vi "wfm_feature clear_adjunct.vi"(8 "error in (no error)":errorcluster, 11 "wfm_feature in":refnum<class "wfm_feature.lvclass">) -> (0 "error out":errorcluster, 3 "wfm_feature out":refnum<class "wfm_feature.lvclass">)   [LabVIEW 2018, in "wfm_feature.lvclass"]
uses:
  wfm_feature.lvclass
  wfm_feature.lvclass/wfm_feature.ctl
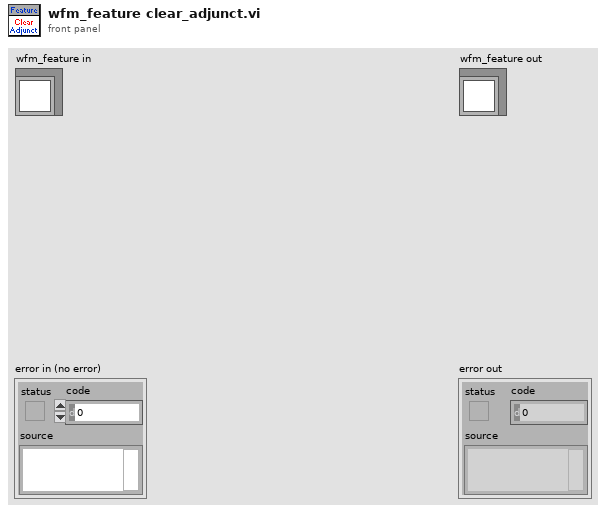
[diagram p1: front panel]
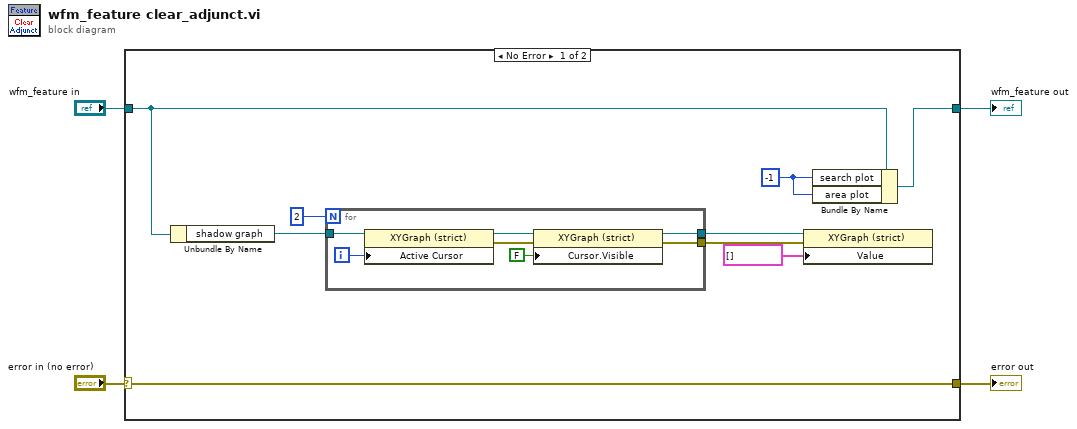
[diagram p0: block diagram]
diagram:
  n1 = case shown="No Error" "error in (no error)" {
    selector: "error in (no error)" -> [w13 w22]
    tunnel: [w13 w22] -> w3
    tunnel: [w5 w21] -> w1
    tunnel: "wfm_feature in" -> [w7 w21]
    frame No Error {
      w6 = -1 ("threshold plot")
      n2 = Unbundle By Name(w7) -> ("shadow graph"=w11:refnum<vi>)
      n3 = for {
        N: 2 -> [_]
        tunnel: w11 -> [w20]
        tunnel: [w15] -> w10
        tunnel: [w14] -> w9
        i -> [w19]
        n4 = property class="XYGraph (strict)"(reference=w20, "Active Cursor"=w19) -> (reference out=w18:refnum<vi>, error out=w17:errorcluster)  [unwired: 1 in]
        n5 = property class="XYGraph (strict)"(reference=w18, error in=w17, "Cursor.Visible"=FALSE) -> (reference out=w15:refnum<vi>, error out=w14:errorcluster)
      }
      n6 = property class="XYGraph (strict)"(reference=w10, error in=w9, "Value"=cluster{"Array":cluster{"X":dbl, "Y":dbl}[]}[] []) -> ()  [unwired: 2 out]
      n7 = Bundle By Name(cluster=w7, "search plot"=w6, "area plot"=w6) -> (w5:refnum<class "wfm_feature.lvclass">)
    }
    frame Error {
    }
  }
  "error out" <- w3
  "wfm_feature out" <- w1
